vi "5_2_take_seeds_give_min.vi"(10 "Map":T1(c390), 11 "element":string) -> (2 "s? t:f 2":i64)   [LabVIEW 2021, in "2023.lvlib"]
uses:
  2023.lvlib
panel:
  out "Numeric 2":i32
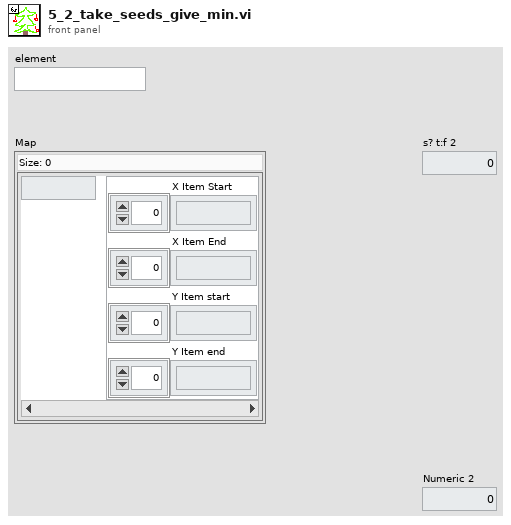
[diagram p1: front panel]
types:
  T1 = map{i32, cluster{"X Item Start":i64[], "X Item End":i64[], "Y Item start":i64[], "Y Item end":i64[]}}
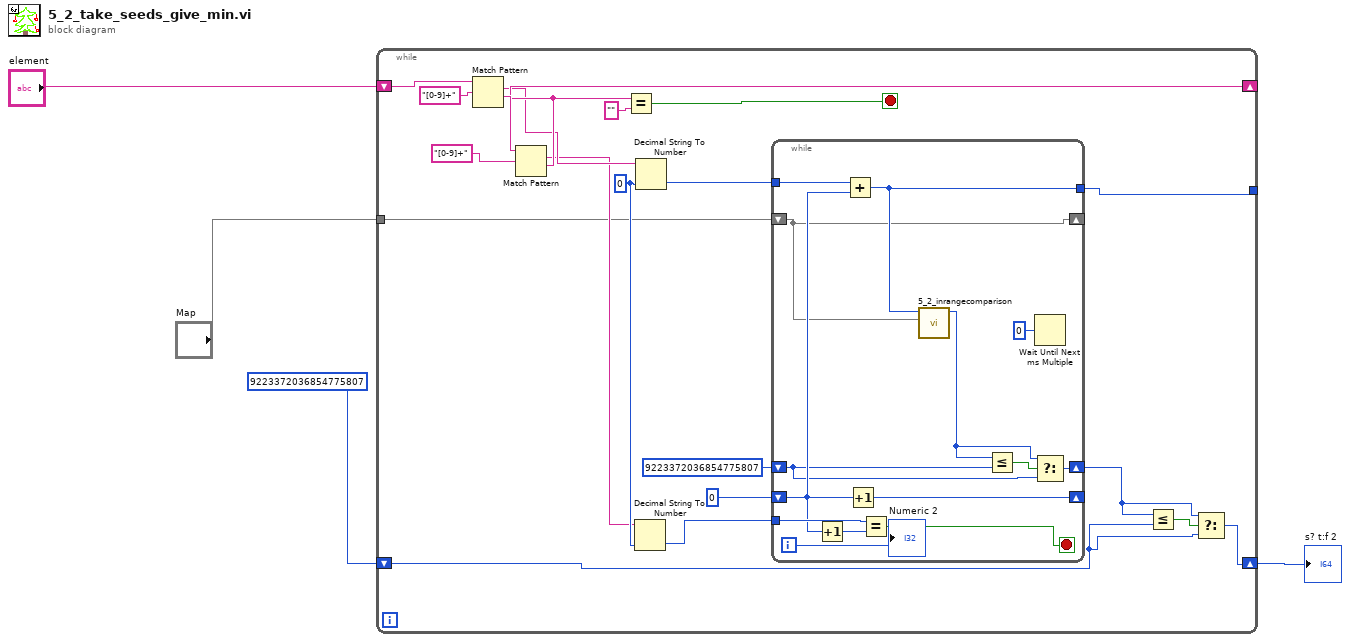
[diagram p0: block diagram]
diagram:
  n1 = while {
    shift-right: [w19] -> _
    shift-left: "element" -> [w24]
    tunnel: [w11] -> _
    tunnel: "Map" -> [w10]
    shift-right: [w6] -> w4
    shift-left: i64 9223372036854775807 ("s? t:f") -> [w7]
    stop <- w21 stop-if-true
    w16 = i64 0 ("element")
    n2 = Match Pattern(string=w24, regular expression="[0-9]+") -> (match substring=w17:string, after substring=w20:string)  [unwired: 1 in, 2 out]
    n3 = Match Pattern(string=w20, regular expression="[0-9]+") -> (match substring=w15:string, after substring=w19:string)  [unwired: 1 in, 2 out]
    n4 = Equal?(x=w19, y="") -> (x = y?=w21:bool)
    n5 = Decimal String To Number(string=w15, default (0L)=w16) -> (number=w13:i64)  [unwired: 1 in, 1 out]
    n6 = Decimal String To Number(string=w17, default (0L)=w16) -> (number=w14:i64)  [unwired: 1 in, 1 out]
    n7 = while {
      tunnel: w14 -> [w37]
      tunnel: w13 -> [w38]
      tunnel: [w29] -> w11
      shift-right: [w34] -> _
      shift-left: i64 0 ("element") -> [w35]
      shift-right: [w28] -> _
      shift-left: w10 -> [w28]
      shift-right: [w30] -> w5
      shift-left: i64 9223372036854775807 ("s? t:f") -> [w31]
      i -> [w27]
      stop <- w36 stop-if-true
      n8 = Increment(x=w35) -> (x+1=w33:i64)
      n9 = Add(x=w37, y=w35) -> (x+y=w29:i64)
      n10 = Increment(x=w35) -> (x+1=w34:i64)
      n11 = Equal?(x=w38, y=w33) -> (x = y?=w36:bool)
      n12 = call "5_2_inrangecomparison.vi"("Map"=w28, "Numeric"=w29) -> ("element"=w26:i64)  [unwired: 9 in]
      n13 = Less Or Equal?(x=w26, y=w31) -> (x <= y?=w32:bool)
      n14 = Wait Until Next ms Multiple(millisecond multiple=u32 0) -> ()  [unwired: 1 out]
      n15 = Select(t=w26, s=w32, f=w31) -> (s? t:f=w30:i64)
      "Numeric 2" <- w27
    }
    n16 = Less Or Equal?(x=w5, y=w7) -> (x <= y?=w8:bool)
    n17 = Select(t=w5, s=w8, f=w7) -> (s? t:f=w6:i64)
  }
  "s? t:f 2" <- w4
